vi "Center VI on Monitor Core.vi"(5 "Make Modal":bool, 7 "Coords (Current Mouse)":T1={"Horizontal"=-1, "Vertical"=-1}, 8 "error in (no error)":errorcluster, 10 "Window Mode (Center on Monitor)":enum16{"Center on Monitor", "Center on Mouse"}(ring), 11 "VI Ref In":refnum<vi>) -> (0 "error out":errorcluster, 3 "VI Ref Out":refnum<vi>)   [LabVIEW 2021, in "Panel Movement Center Maximize.lvlib"]
doc: "-----\nHooovahh\n(Brian Hoover)"
uses:
  Panel Movement Center Maximize.lvlib
  <vilib>/Utility/miscctls.llb/LVPoint32TypeDef.ctl
  <vilib>/Utility/miscctls.llb/LVRectTypeDef.ctl
  System.Windows.Forms
  System.Drawing
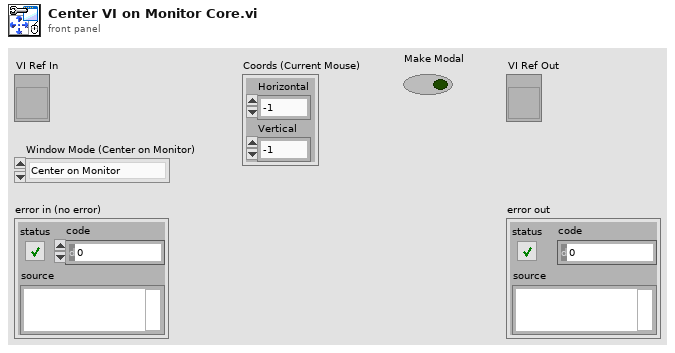
[diagram p1: front panel]
types:
  T1 = typedef "LVPoint32TypeDef.ctl" = cluster{"Horizontal":i32, "Vertical":i32}
  T2 = enum32{"Invalid", "Default", "Floating", "Floating/Auto-Hide", "Modal"}
  T3 = typedef "LVRectTypeDef.ctl" = cluster{"Left":i16, "Top":i16, "Right":i16, "Bottom":i16}
  T4 = typedef "LVBoundsTypeDef.ctl" = cluster{"Width":u32, "Height":u32}
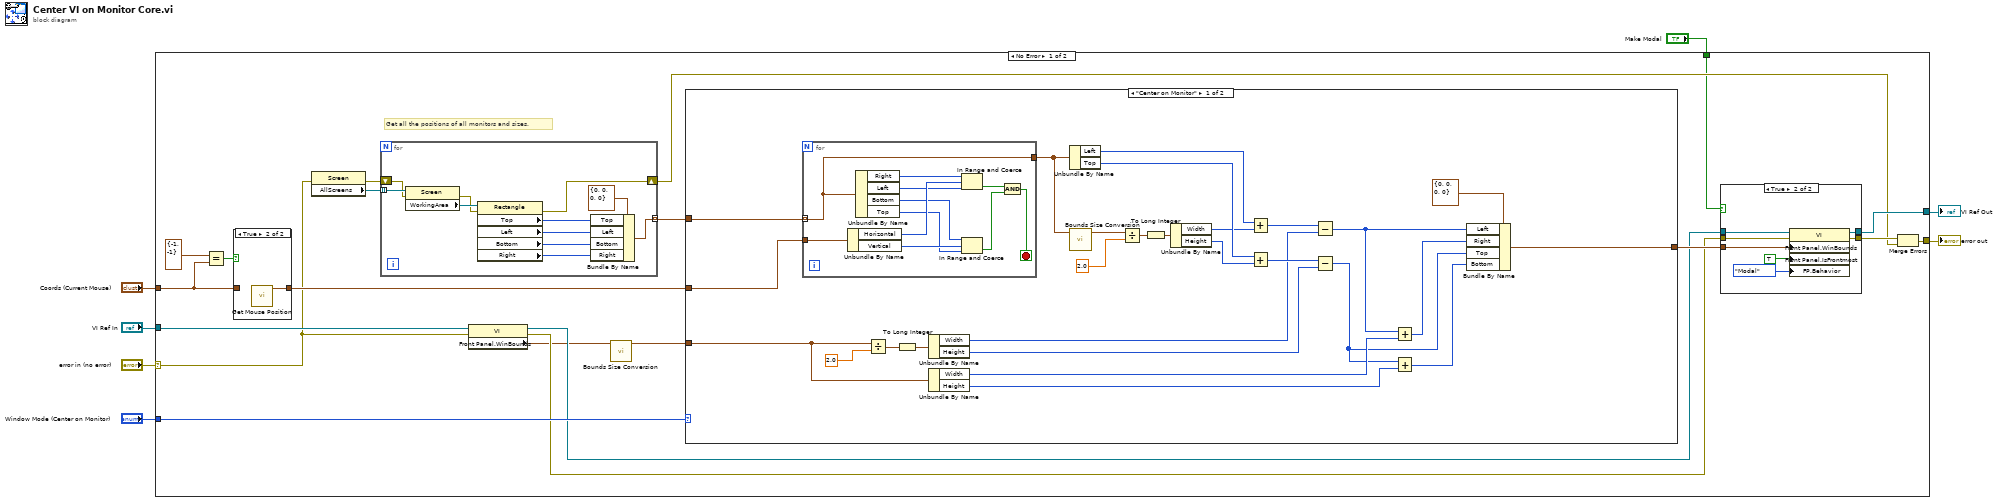
[diagram p0: block diagram]
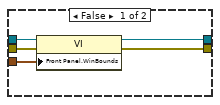
[diagram p2: hidden frame]
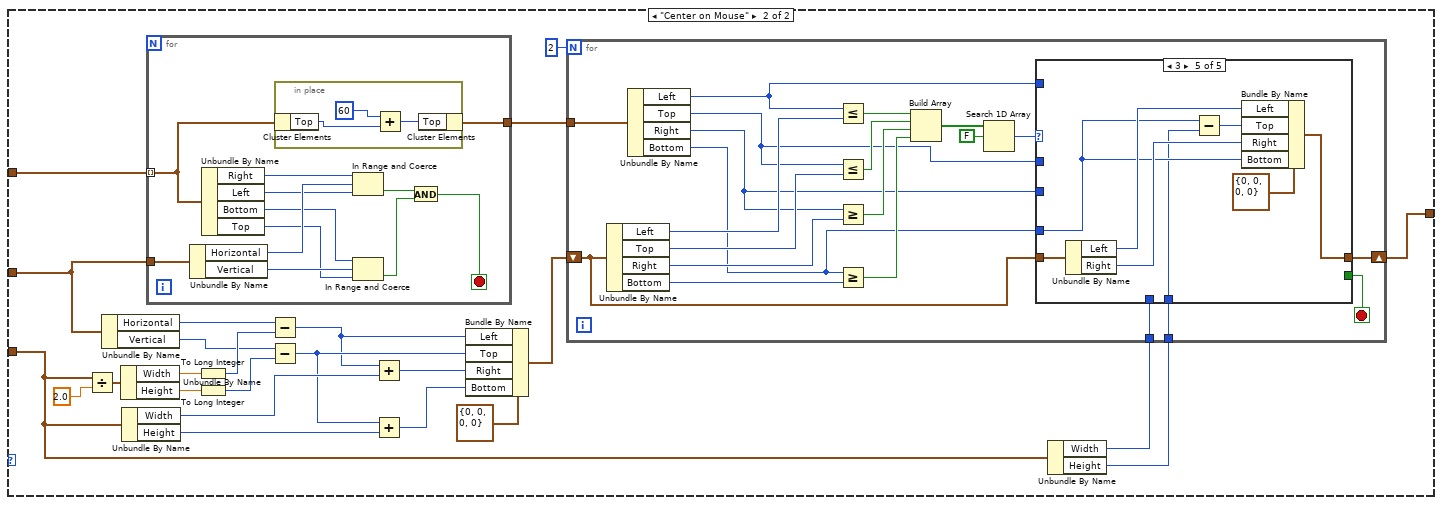
[diagram p3: hidden frame]
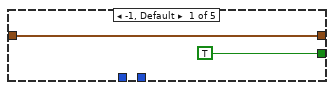
[diagram p4: hidden frame]
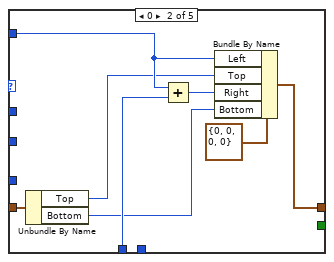
[diagram p5: hidden frame]
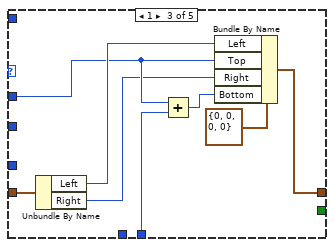
[diagram p6: hidden frame]
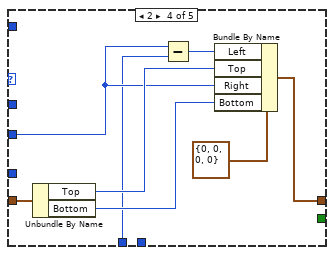
[diagram p7: hidden frame]
diagram:
  n1 = case shown="No Error" "error in (no error)" {
    selector: "error in (no error)" -> [w11 w186]
    tunnel: "Window Mode (Center on Monitor)" -> [w27 _]
    tunnel: "Coords (Current Mouse)" -> [w23 _]
    tunnel: [w22 w185] -> w5
    tunnel: "VI Ref In" -> [w18 w185]
    tunnel: [w10 w186] -> w2
    tunnel: "Make Modal" -> [w8 _]
    frame No Error {
      # "Get all the positions of all monitors and sizes."
      n2 = Equal?(x=T1 {"Horizontal"=-1, "Vertical"=-1}, y=w23) -> (x = y?=w13:bool)
      n3 = case shown="True" w13 {
        tunnel: w23 -> [w183 _]
        tunnel: [w183 w184] -> w24
        frame False {
        }
        frame True {
          n4 = call "Get Mouse Position.vi"() -> ("Mouse Position"=w184:cluster{"Horizontal":i32, "Vertical":i32})  [unwired: 10 in, 1 out]
        }
      }
      n5 = property class="Screen"(error in=w11) -> (error out=w16:errorcluster, "AllScreens"=w15:refnum<k24>[])  [unwired: 1 in, 1 out]
      n6 = for {
        tunnel: w15 -> [w180] mode=indexing
        shift-right: [w178] -> w9
        shift-left: w16 -> [w179]
        tunnel: [w173] -> w17 mode=indexing
        n7 = property class="Screen"(reference=w180, error in=w179) -> (error out=w181:errorcluster, "WorkingArea"=w182:refnum<k24>)  [unwired: 1 out]
        n8 = property class="Rectangle"(reference=w182, error in=w181) -> (error out=w178:errorcluster, "Top"=w172:i32, "Left"=w176:i32, "Bottom"=w175:i32, "Right"=w174:i32)  [unwired: 1 out]
        n9 = Bundle By Name(cluster=T3 {"Left"=0, "Top"=0, "Right"=0, "Bottom"=0} ("Front Panel Window:Panel Bounds"), "Top"=w172, "Left"=w176, "Bottom"=w175, "Right"=w174) -> (w173:T3)
      }
      n10 = property class="VI"(reference=w18, error in=w11) -> (reference out=w19:refnum<vi>, error out=w20:errorcluster, "Front Panel.WinBounds"=w14:T3)
      n11 = call "Bounds Size Conversion.vi"("Bounds"=w14) -> ("Size Out"=w26:T4)  [unwired: 9 in, 1 out]
      n12 = case shown="\"Center on Monitor\"" w27 {
        tunnel: w17 -> [w64 w98]
        tunnel: w24 -> [w63 w83]
        tunnel: [w61 w99] -> w25
        tunnel: w26 -> [w58 w78]
        frame "Center on Monitor" {
          n13 = for {
            tunnel: w63 -> [w77]
            tunnel: w64 -> [w67] mode=indexing
            tunnel: [w67] -> w53
            stop <- w68 stop-if-true
            n14 = Unbundle By Name(w77) -> ("Horizontal"=w76:i32, "Vertical"=w74:i32)
            n15 = Unbundle By Name(w67) -> ("Right"=w75:i16, "Left"=w73:i16, "Bottom"=w72:i16, "Top"=w71:i16)
            n16 = In Range and Coerce(upper limit=w75, x=w76, lower limit=w73) -> (In Range?=w70:bool)  [unwired: 1 out]
            n17 = In Range and Coerce(upper limit=w72, x=w74, lower limit=w71) -> (In Range?=w69:bool)  [unwired: 1 out]
            n18 = And(x=w70, y=w69) -> (x .and. y?=w68:bool)
          }
          n19 = Divide(x=w58, y=2.0) -> (x/y=w65:cluster{"Width":dbl, "Height":dbl})
          n20 = To Long Integer(number=w65) -> (32bit integer=w42:cluster{"Width":i32, "Height":i32})
          n21 = Unbundle By Name(w42) -> ("Width"=w41:i32, "Height"=w40:i32)
          n22 = Unbundle By Name(w58) -> ("Width"=w57:u32, "Height"=w55:u32)
          n23 = Unbundle By Name(w53) -> ("Left"=w60:i16, "Top"=w59:i16)
          n24 = call "Bounds Size Conversion.vi"("Bounds"=w53) -> ("Size Out"=w52:T4)  [unwired: 9 in, 1 out]
          n25 = Divide(x=w52, y=2.0) -> (x/y=w45:cluster{"Width":dbl, "Height":dbl})
          n26 = To Long Integer(number=w45) -> (32bit integer=w43:cluster{"Width":i32, "Height":i32})
          n27 = Unbundle By Name(w43) -> ("Width"=w51:i32, "Height"=w50:i32)
          n28 = Add(x=w60, y=w51) -> (x+y=w49:i32)
          n29 = Add(x=w59, y=w50) -> (x+y=w48:i32)
          n30 = Subtract(x=w49, y=w41) -> (x-y=w47:i32)
          n31 = Subtract(x=w48, y=w40) -> (x-y=w46:i32)
          n32 = Add(x=w47, y=w57) -> (x+y=w56:u32)
          n33 = Add(x=w46, y=w55) -> (x+y=w54:u32)
          n34 = Bundle By Name(cluster=T3 {"Left"=0, "Top"=0, "Right"=0, "Bottom"=0} ("Front Panel Window:Window Bounds"), "Left"=w47, "Right"=w56, "Top"=w46, "Bottom"=w54) -> (w61:T3)
        }
        frame "Center on Mouse" {
          n35 = Divide(x=w78, y=2.0) -> (x/y=w85:cluster{"Width":dbl, "Height":dbl})
          n36 = Unbundle By Name(w83) -> ("Horizontal"=w86:i32, "Vertical"=w87:i32)
          n37 = Unbundle By Name(w85) -> ("Width"=w90:dbl, "Height"=w88:dbl)
          n38 = Unbundle By Name(w78) -> ("Width"=w96:u32, "Height"=w97:u32)
          n39 = for {
            tunnel: w83 -> [w168]
            tunnel: [w158] -> w101
            tunnel: w98 -> [w157] mode=indexing
            stop <- w159 stop-if-true
            n40 = Unbundle By Name(w168) -> ("Horizontal"=w167:i32, "Vertical"=w165:i32)
            n41 = Unbundle By Name(w157) -> ("Right"=w166:i16, "Left"=w164:i16, "Bottom"=w163:i16, "Top"=w162:i16)
            n42 = in-place {
              n43 = in-place-cluster #1(w157) -> ("Top"=w171:i16)
              n44 = Add(x=60, y=w171) -> (x+y=w170:i32)
              n45 = in-place-cluster #1("Top"=w170) -> (w158:T3)
            }
            n46 = In Range and Coerce(upper limit=w166, x=w167, lower limit=w164) -> (In Range?=w161:bool)  [unwired: 1 out]
            n47 = In Range and Coerce(upper limit=w163, x=w165, lower limit=w162) -> (In Range?=w160:bool)  [unwired: 1 out]
            n48 = And(x=w161, y=w160) -> (x .and. y?=w159:bool)
          }
          n49 = To Long Integer(number=w90) -> (32bit integer=w92:i32)
          n50 = To Long Integer(number=w88) -> (32bit integer=w94:i32)
          n51 = Subtract(x=w86, y=w92) -> (x-y=w89:i32)
          n52 = Subtract(x=w87, y=w94) -> (x-y=w93:i32)
          n53 = Add(x=w89, y=w96) -> (x+y=w91:u32)
          n54 = Add(x=w93, y=w97) -> (x+y=w95:u32)
          n55 = Bundle By Name(cluster=T3 {"Left"=0, "Top"=0, "Right"=0, "Bottom"=0} ("Front Panel Window:Panel Bounds"), "Left"=w89, "Top"=w93, "Right"=w91, "Bottom"=w95) -> (w81:T3)
          n56 = Unbundle By Name(w78) -> ("Width"=w80:u32, "Height"=w79:u32)
          n57 = for {
            N: 2 -> [_]
            tunnel: w101 -> [w122]
            shift-right: [w107] -> w99
            shift-left: w81 -> [w106]
            tunnel: w80 -> [w109]
            tunnel: w79 -> [w108]
            stop <- w112 stop-if-true
            n58 = Unbundle By Name(w106) -> ("Left"=w121:i16, "Top"=w110:i16, "Right"=w120:i16, "Bottom"=w119:i16)
            n59 = Unbundle By Name(w122) -> ("Left"=w111:i16, "Top"=w105:i16, "Right"=w104:i16, "Bottom"=w103:i16)
            n60 = Less Or Equal?(x=w111, y=w121) -> (x <= y?=w118:bool)
            n61 = Less Or Equal?(x=w105, y=w110) -> (x <= y?=w117:bool)
            n62 = Greater Or Equal?(x=w104, y=w120) -> (x >= y?=w116:bool)
            n63 = Greater Or Equal?(x=w103, y=w119) -> (x >= y?=w115:bool)
            n64 = Build Array(w118, w117, w116, w115) -> (w114:bool[])
            n65 = Search 1D Array(1D array=w114, element=FALSE) -> (index of element=w102:i32)  [unwired: 1 in]
            n66 = case shown="3" w102 {
              tunnel: [TRUE _ _ _ _] -> w112
              tunnel: w111 -> [_ w130 _ _ _]
              tunnel: w109 -> [_ w129 _ w142 _]
              tunnel: w108 -> [_ _ w138 _ w150]
              tunnel: [w123 w128 w137 w147 w155] -> w107
              tunnel: w106 -> [w123 w127 w136 w146 w154]
              tunnel: w105 -> [_ _ w134 _ _]
              tunnel: w104 -> [_ _ _ w143 _]
              tunnel: w103 -> [_ _ _ _ w151]
              frame -1, Default {
              }
              frame 0 {
                n67 = Unbundle By Name(w127) -> ("Top"=w126:i16, "Bottom"=w125:i16)
                n68 = Add(x=w130, y=w129) -> (x+y=w132:u32)
                n69 = Bundle By Name(cluster=T3 {"Left"=0, "Top"=0, "Right"=0, "Bottom"=0} ("Front Panel Window:Panel Bounds"), "Left"=w130, "Top"=w126, "Right"=w132, "Bottom"=w125) -> (w128:T3)
              }
              frame 1 {
                n70 = Unbundle By Name(w136) -> ("Left"=w135:i16, "Right"=w133:i16)
                n71 = Add(x=w134, y=w138) -> (x+y=w140:u32)
                n72 = Bundle By Name(cluster=T3 {"Left"=0, "Top"=0, "Right"=0, "Bottom"=0} ("Front Panel Window:Panel Bounds"), "Left"=w135, "Top"=w134, "Right"=w133, "Bottom"=w140) -> (w137:T3)
              }
              frame 2 {
                n73 = Unbundle By Name(w146) -> ("Top"=w145:i16, "Bottom"=w144:i16)
                n74 = Subtract(x=w143, y=w142) -> (x-y=w141:u32)
                n75 = Bundle By Name(cluster=T3 {"Left"=0, "Top"=0, "Right"=0, "Bottom"=0} ("Front Panel Window:Panel Bounds"), "Left"=w141, "Top"=w145, "Right"=w143, "Bottom"=w144) -> (w147:T3)
              }
              frame 3 {
                n76 = Unbundle By Name(w154) -> ("Left"=w153:i16, "Right"=w152:i16)
                n77 = Subtract(x=w151, y=w150) -> (x-y=w149:u32)
                n78 = Bundle By Name(cluster=T3 {"Left"=0, "Top"=0, "Right"=0, "Bottom"=0} ("Front Panel Window:Panel Bounds"), "Left"=w153, "Top"=w149, "Right"=w152, "Bottom"=w151) -> (w155:T3)
              }
            }
          }
        }
      }
      n79 = case shown="True" w8 {
        tunnel: w25 -> [w32 w35]
        tunnel: [w31 w34] -> w22
        tunnel: [w30 w33] -> w21
        tunnel: w20 -> [w29 w36]
        tunnel: w19 -> [w28 w37]
        frame False {
          n80 = property class="VI"(reference=w28, error in=w29, "Front Panel.WinBounds"=w32) -> (reference out=w31:refnum<vi>, error out=w30:errorcluster)
        }
        frame True {
          n81 = property class="VI"(reference=w37, error in=w36, "Front Panel.WinBounds"=w35, "Front Panel.IsFrontmost"=TRUE ("Front Panel Window:Is Frontmost"), "FP.Behavior"=T2."Modal" ("Front Panel Window:Behavior")) -> (reference out=w34:refnum<vi>, error out=w33:errorcluster)
        }
      }
      n82 = Merge Errors(w21, w9) -> (w10:errorcluster)
    }
    frame Error {
    }
  }
  "VI Ref Out" <- w5
  "error out" <- w2
